vi "GreaterOrEqual.vi"(0 "VI Reference In":refnum<vi>, 1 "Test Label":string, 2 "delimiter (>>)":string=">>", 3 "Assert Only? (F)":bool, 5 "Control Path":string, 7 "Control Value":variant, 11 "Error In":errorcluster, 12 "Assert Interval(10 ms)":u32=10, 13 "Timeout(5 sec)":dbl=5.0) -> (4 "VI Reference Out":refnum<vi>, 6 "Test Value":variant, 15 "Error Out":errorcluster)   [LabVIEW 2016, in "Drona.lvlib" / "AssertControlValue.lvlib"]
doc: "Asserts if the value of control is greater or equal to the input value.\n\nThe input control name is given as a string , incase of path, use delimiters inbetween the path.\nThis VI gets the value of the control, untill the value is greater or equal to the input value."
uses:
  AssertControlValue.lvlib
  Get/GetControlRef/GetControlRefByPath.vi
  <vilib>/addons/_JKI Toolkits/Caraya/classes/Assert/Assert Greater Or Equal_Variant.vi
  <vilib>/addons/_JKI Toolkits/Caraya/classes/Assert/Assert.lvclass
  Get/GetControlRef/GetControlRef.lvlib
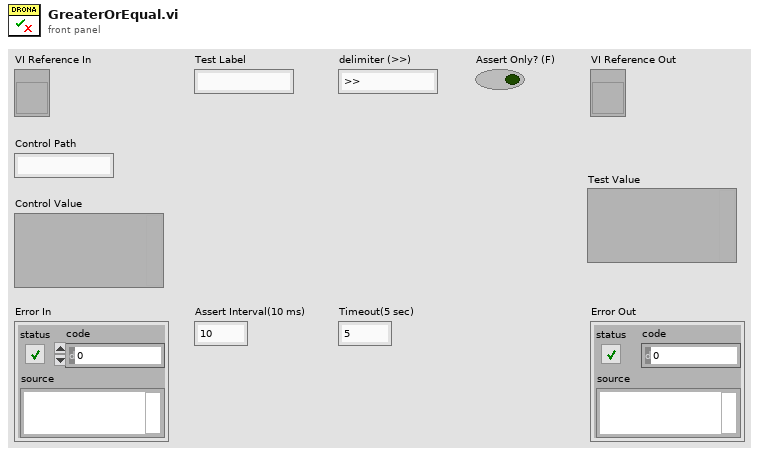
[diagram p1: front panel]
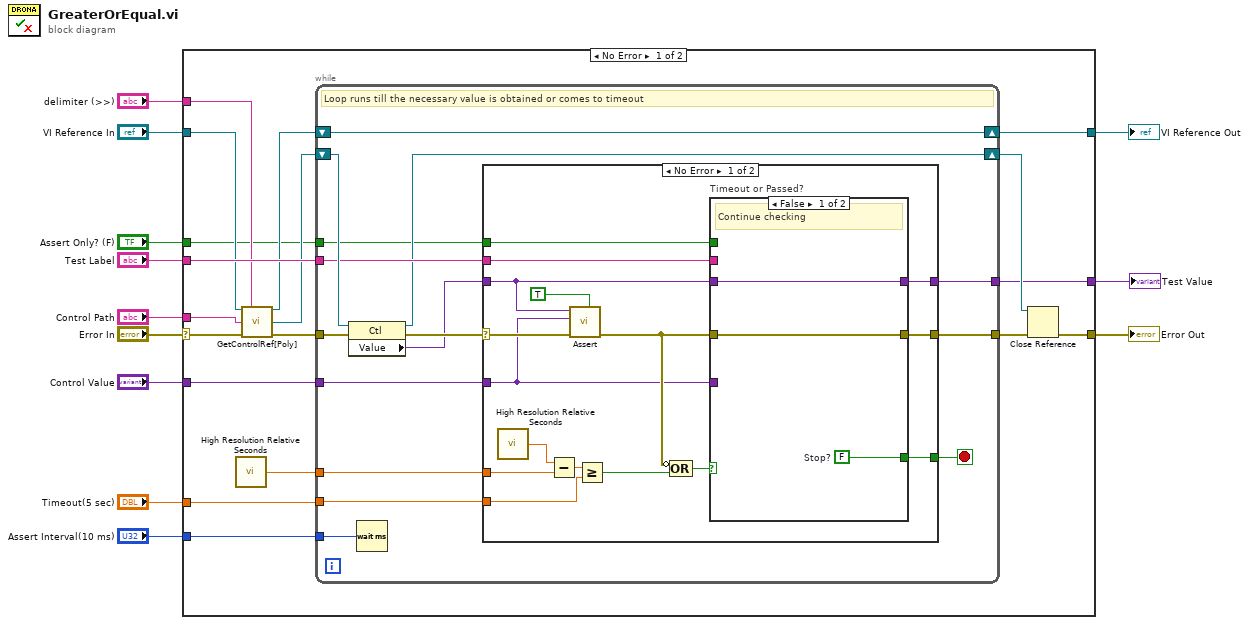
[diagram p0: block diagram]
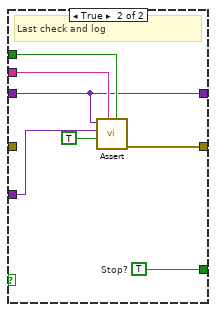
[diagram p2: hidden frame]
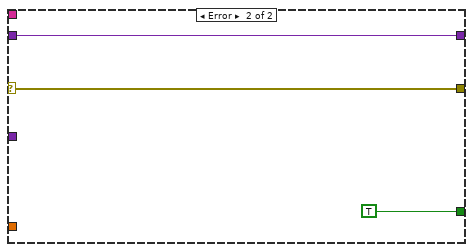
[diagram p3: hidden frame]
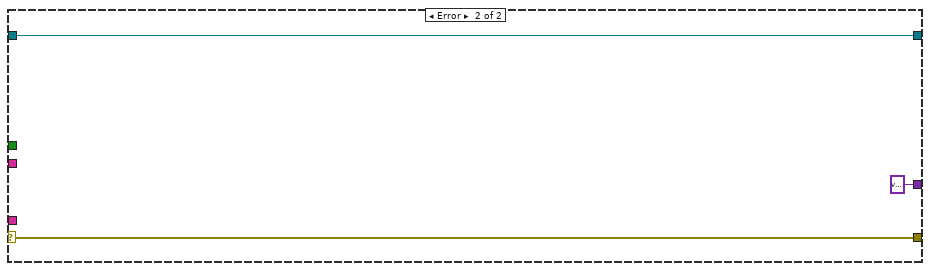
[diagram p4: hidden frame]
diagram:
  n1 = case shown="No Error" "Error In" {
    selector: "Error In" -> [w24 w77]
    tunnel: "Timeout(5 sec)" -> [w30 _]
    tunnel: [w29 w76] -> w11
    tunnel: "Control Value" -> [w28 _]
    tunnel: [w17 w77] -> w9
    tunnel: "Assert Interval(10 ms)" -> [w26 _]
    tunnel: "Test Label" -> [w25 _]
    tunnel: "VI Reference In" -> [w23 w76]
    tunnel: "Control Path" -> [w22 _]
    tunnel: "delimiter (>>)" -> [w15 _]
    tunnel: "Assert Only? (F)" -> [w14 _]
    tunnel: [w13 variant ("Value")] -> w1
    frame No Error {
      n2 = call <vilib>:"High Resolution Relative Seconds.vi"() -> ("relative seconds"=w21:dbl)
      n3 = call-poly "GetControlRef[Poly].vi"("VI Reference In"=w23, "delimiter (>>)"=w15, "Control Path"=w22, "error In"=w24) -> ("VI Reference Out"=w19:refnum<vi>, "Ctl Refnum"=w18:refnum<vi>, "error out"=w20:errorcluster)  [unwired: 9 in]
      n4 = while {
        tunnel: w28 -> [w39]
        tunnel: w30 -> [w44]
        tunnel: w21 -> [w45]
        tunnel: w20 -> [w38]
        tunnel: [w42] -> w27
        tunnel: w26 -> [w40]
        tunnel: w25 -> [w34]
        shift-right: [w36] -> w29
        shift-left: w19 -> [w36]
        shift-right: [w33] -> w16
        shift-left: w18 -> [w37]
        tunnel: w14 -> [w32]
        tunnel: [w31] -> w13
        stop <- w43 stop-if-true
        # "Loop runs till the necessary value is obtained or comes to timeout"
        n5 = property class="Ctl"(reference=w37, error in=w38) -> (reference out=w33:refnum<vi>, error out=w41:errorcluster, "Value"=w35:variant)
        n6 = Wait (ms)(milliseconds to wait=w40) -> ()  [unwired: 1 out]
        n7 = case shown="No Error" w41 {
          selector: w41 -> [w57 w74]
          tunnel: w45 -> [w61 _]
          tunnel: w44 -> [w58 _]
          tunnel: [w48 TRUE] -> w43
          tunnel: [w49 w74] -> w42
          tunnel: w39 -> [w50 _]
          tunnel: w35 -> [w51 w72]
          tunnel: w34 -> [w56 _]
          tunnel: w32 -> [w47 _]
          tunnel: [w46 w72] -> w31
          frame No Error {
            n8 = call <vilib>:"High Resolution Relative Seconds.vi"() -> ("relative seconds"=w60:dbl)
            n9 = Subtract(x=w60, y=w61) -> (x-y=w59:dbl)
            n10 = call-poly <vilib>:"Assert.vi"("Assert Only? (F)"=TRUE, "error in (no error)"=w57, "Y"=w50, "X"=w51) -> ("error out"=w54:errorcluster)  [unwired: 7 in]
            n11 = Greater Or Equal?(x=w59, y=w58) -> (x >= y?=w55:bool)
            n12 = Compound Arithmetic op=OR(invert w54, w55) -> (w53:bool)
            n13 = case "Timeout or Passed?" shown="False" w53 {
              tunnel: w54 -> [w64 _]
              tunnel: w50 -> [_ w70]
              tunnel: w51 -> [w62 w65]
              tunnel: w56 -> [_ w71]
              tunnel: [w64 w69] -> w49
              tunnel: [w63 w68] -> w48
              tunnel: w47 -> [_ w66]
              tunnel: [w62 w65] -> w46
              frame False {
                w63 = FALSE  # Stop?
                # "Continue checking"
              }
              frame True {
                w68 = TRUE  # Stop?
                # "Last check and log"
                n14 = call-poly <vilib>:"Assert.vi"("Assert Only? (F)"=w66, "Label"=w71, "Register with caller test (F)"=TRUE, "Y"=w70, "X"=w65) -> ("error out"=w69:errorcluster)  [unwired: 6 in]
              }
            }
          }
          frame Error {
          }
        }
      }
      n15 = Close Reference(reference=w16, error in (no error)=w27) -> (error out=w17:errorcluster)
    }
    frame Error {
    }
  }
  "Error Out" <- w9
  "VI Reference Out" <- w11
  "Test Value" <- w1
